vi "Add Sensor.vi"(7 "SensorInfo":T1={"Sensor Name"="", "Protocol"=enum."UDP", "Network port"=48185, "# Culled Objects"=1, "PlayerID"=1, "MM Data"=[]}, 8 "error in (no error)":errorcluster, 11 "Item Ref in":T7 format="%.0x") -> (0 "error out (no error)":errorcluster)   [LabVIEW 2018, in "Vires VTD System Explorer.lvlib"]
uses:
  Vires VTD System Explorer.lvlib
  <vilib>/NI Veristand/Custom Device API/Custom Device Item Ref.ctl
  Shared/SensorInfo.ctl
  Shared/Sensor Name.ctl
  Shared/Protocol.ctl
  MM/MM Data.ctl
  MM/MM Objects.ctl
  MM/MM Object.ctl
  <vilib>/NI Veristand/Custom Device API/Custom Device Channel.ctl
  <vilib>/NI Veristand/Custom Device API/Custom Device Channel Type.ctl
  Shared/Constants.vi
  <vilib>/NI Veristand/Custom Device API/Set Item Property (Variant).vi
  <vilib>/NI Veristand/Custom Device API/Custom Device API.lvlib
  Shared/Vires VTD Shared.lvlib
  MM/MM.lvlib
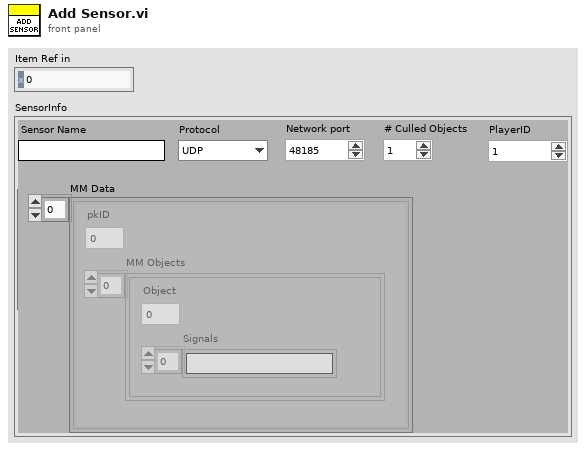
[diagram p1: front panel]
types:
  T1 = typedef "Vires VTD Shared.lvlib/SensorInfo.ctl" = cluster{"Sensor Name":T2, "Protocol":T3, "Network port":i32, "# Culled Objects":i32, "PlayerID":u8, "MM Data":T4}
  T2 = typedef "Vires VTD Shared.lvlib/Sensor Name.ctl" = string
  T3 = typedef "Vires VTD Shared.lvlib/Protocol.ctl" = enum16{"UDP", "TCP"}
  T4 = typedef "Vires VTD Shared.lvlib/MM Data.ctl" = T5[]
  T5 = typedef "MM.lvlib/MM Objects.ctl" = cluster{"pkID":i32, "MM Objects":T6[]}
  T6 = typedef "MM.lvlib/MM Object.ctl" = cluster{"Object":i32, "Signals":string[]}
  T7 = typedef "Custom Device API.lvlib/Custom Device Item Ref.ctl" = u64
  T8 = typedef "Custom Device API.lvlib/Custom Device Channel.ctl" = cluster{"Type":T9, "Units":string, "Default Value":dbl, "Faultable":bool, "Scalable":bool}
  T9 = typedef "Custom Device API.lvlib/Custom Device Channel Type.ctl" = enum16{"Input", "Output"}
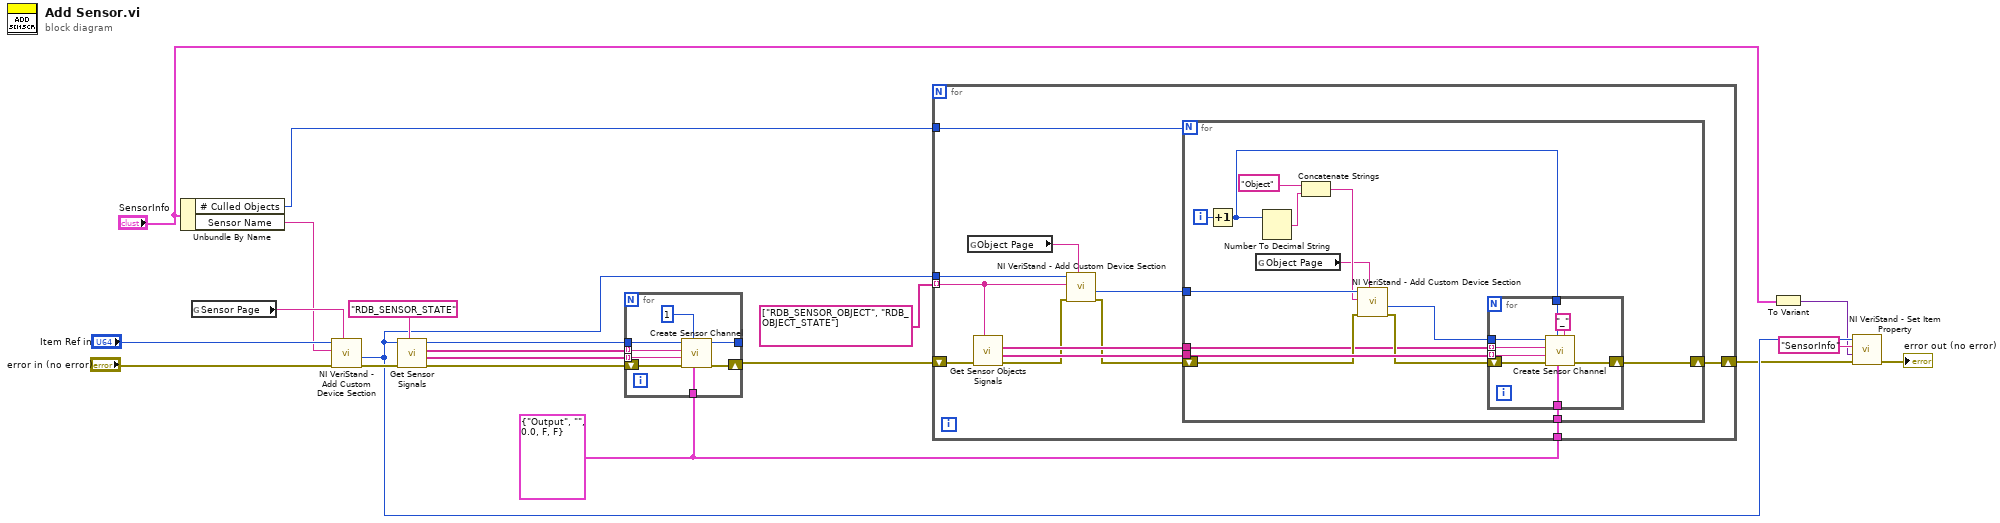
[diagram p0: block diagram]
diagram:
  w9 = T8 {"Type"=enum."Output", "Units"="", "Default Value"=0.0, "Faultable"=FALSE, "Scalable"=FALSE} ("Channel")
  n1 = Unbundle By Name("SensorInfo") -> ("# Culled Objects"=w11:i32, "Sensor Name"=w10:T2)
  n2 = global read "Constants.vi" "Sensor Page"() -> (w13:string)
  n3 = call <vilib>:"NI VeriStand - Add Custom Device Section.vi"("GUID (Default Section)"=w13, "error in (no error)"="error in (no error)", "Section Name"=w10, "Parent Ref in"="Item Ref in") -> ("error out"=w16:errorcluster, "Section Ptr"=w6:T7)  [unwired: 4 in, 2 out]
  n4 = call "Get Sensor Signals.vi"("Filter Cluster"="RDB_SENSOR_STATE", "error in (no error)"=w16, "Item Ref in"=w6) -> ("error out (no error)"=w17:errorcluster, "Sensor Signals"=w8:string[], "Sensor Names"=w15:string[], "Item Ref out"=w14:T7)  [unwired: 5 in]
  n5 = for {
    shift-right: [w28] -> w12
    shift-left: w17 -> [w27]
    tunnel: w15 -> [w24] mode=indexing
    tunnel: w14 -> [w25]
    tunnel: w9 -> [w26]
    tunnel: w8 -> [w23] mode=indexing
    tunnel: [w22] -> _
    n6 = call "Create Sensor Channel.vi"("Channel"=w26, "Object"=1, "error in (no error)"=w27, "RDB Signalname"=w23, "RDB Receive Objects"=w24, "Item Ref in"=w25) -> ("error out"=w28:errorcluster, "pkid"=w22:u32)  [unwired: 4 in]
  }
  n7 = for {
    tunnel: w11 -> [w38]
    tunnel: w9 -> [w37]
    tunnel: w6 -> [w34]
    shift-right: [w39] -> w5
    shift-left: w12 -> [w40]
    tunnel: string[] ["RDB_SENSOR_OBJECT", "RDB_OBJECT_STATE"] -> [w31] mode=indexing
    n8 = global read "Constants.vi" "Object Page"() -> (w30:string)
    n9 = call "Get Sensor Objects Signals.vi"("Filter Cluster"=w31, "error in (no error)"=w40) -> ("error out (no error)"=w33:errorcluster, "Sensor Signals"=w36:string[], "Sensor Names"=w35:string[])  [unwired: 7 in]
    n10 = call <vilib>:"NI VeriStand - Add Custom Device Section.vi"("GUID (Default Section)"=w30, "error in (no error)"=w33, "Section Name"=w31, "Parent Ref in"=w34) -> ("error out"=w32:errorcluster, "Section Ptr"=w29:T7)  [unwired: 4 in, 2 out]
    n11 = for {
      N: w38 -> [_]
      shift-right: [w54] -> w39
      shift-left: w32 -> [w51]
      tunnel: w37 -> [w53]
      tunnel: w36 -> [w52]
      tunnel: w29 -> [w49]
      tunnel: w35 -> [w42]
      i -> [w46]
      n12 = Increment(x=w46) -> (x+1=w41:i32)
      n13 = global read "Constants.vi" "Object Page"() -> (w43:string)
      n14 = Number To Decimal String(number=w41) -> (decimal integer string=w45:string)  [unwired: 1 in]
      n15 = Concatenate Strings("Object" ("Section Name"), w45) -> (w44:string)
      n16 = call <vilib>:"NI VeriStand - Add Custom Device Section.vi"("GUID (Default Section)"=w43, "error in (no error)"=w51, "Section Name"=w44, "Parent Ref in"=w49) -> ("error out"=w50:errorcluster, "Section Ptr"=w48:T7)  [unwired: 4 in, 2 out]
      n17 = for {
        tunnel: w53 -> [w56]
        shift-right: [w62] -> w54
        shift-left: w50 -> [w61]
        tunnel: w48 -> [w60]
        tunnel: w41 -> [w59]
        tunnel: w52 -> [w55] mode=indexing
        tunnel: w42 -> [w58] mode=indexing
        n18 = call "Create Sensor Channel.vi"("regular expression"="_", "Channel"=w56, "Object"=w59, "error in (no error)"=w61, "RDB Signalname"=w55, "RDB Receive Objects"=w58, "Item Ref in"=w60) -> ("error out"=w62:errorcluster)  [unwired: 3 in, 1 out]
      }
    }
  }
  n19 = To Variant(anything="SensorInfo") -> (Variant=w2:variant)
  n20 = call-poly <vilib>:"NI VeriStand - Set Item Property.vi"("error in (no error)"=w5, "Value"=w2, "Property Name"="SensorInfo" ("String"), "Item Ref in"=w6) -> ("error out"=→"error out (no error)":errorcluster)  [unwired: 5 in, 2 out]
